vi "SVPO Convert to Even Angle Signal.vi"   [LabVIEW 2017, in "SoundVib_OrderTracking.lvlib"]
doc: "Converts an even-time-spaced scaled signal to an even-angle-spaced signal by resampling the acquired signal. The output signal is synchronous to the rotational speed with a constant number of samples per revolution. Use this VI on embedded targets that have limited computational resources. Wire data to the <B>scaled signal [EU]</B> input to determine the polymorphic instance to use or manually select the instance."
uses:
  <vilib>/addons/Sound and Vibration/Order Analysis/Resample Order Tracking/SoundVib_OrderTracking.lvlib
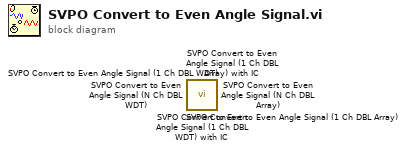
[diagram p0: block diagram]
diagram:
  n1 = call <vilib>:"SVPO Convert to Even Angle Signal (1 Ch DBL WDT) with IC.vi"() -> ()  [unwired: 13 in, 3 out]
  n2 = call <vilib>:"SVPO Convert to Even Angle Signal (1 Ch DBL Array) with IC.vi"() -> ()  [unwired: 13 in, 3 out]
  n3 = call <vilib>:"SVPO Convert to Even Angle Signal (N Ch DBL WDT).vi"() -> ()  [unwired: 14 in, 2 out]
  n4 = call <vilib>:"SVPO Convert to Even Angle Signal (N Ch DBL Array).vi"() -> ()  [unwired: 14 in, 2 out]
  n5 = call <vilib>:"SVPO Convert to Even Angle Signal (1 Ch DBL WDT).vi"() -> ()  [unwired: 14 in, 2 out]
  n6 = call <vilib>:"SVPO Convert to Even Angle Signal (1 Ch DBL Array).vi"() -> ()  [unwired: 14 in, 2 out]
